vi "AIT 1553 - Read FIFOs.vi"(5 "Bus Section":T1, 7 "Mode":T2, 8 "error in (no error)":errorcluster, 11 "RT Data in":T3 {"Acyclic Frame Refs" format="%.0x"; "Label Transfer Config"."Block Data Refs"."Data Reference" format="%.0x"; "Status Config"."HWOut Dur Ref" format="%.0x"; "Status Config"."HWIn Dur Ref" format="%.0x"; "Status Config"."HWOut Count Ref" format="%.0x"; "Status Config"."HWIn Count Ref" format="%.0x"; "Status Config"."Error Data Ref" format="%.0x"; "HWOutput Channels"."Message Settings"."Driver Data"."First Word" min=8 max=31; "HWOutput Channels"."Message Settings"."Driver Data"."Num Bits" min=1 max=32; "HWOutput Channels"."Message Settings"."Driver Data"."Start Bit" min=8 max=31; "HWOutput Channels"."Message Settings"."Block Data Refs"."Data Reference" format="%.0x"; "HWInput Channels"."Message Settings"."Driver Data"."First Word" min=8 max=31; "HWInput Channels"."Message Settings"."Driver Data"."Num Bits" min=1 max=32; "HWInput Channels"."Message Settings"."Driver Data"."Start Bit" min=8 max=31; "HWInput Channels"."Message Settings"."Block Data Refs"."Data Reference" format="%.0x"}) -> (0 "error out":errorcluster, 3 "RT Data out":T3 {"Acyclic Frame Refs" format="%.0x"; "Label Transfer Config"."Block Data Refs"."Data Reference" format="%.0x"; "Status Config"."HWOut Dur Ref" format="%.0x"; "Status Config"."HWIn Dur Ref" format="%.0x"; "Status Config"."HWOut Count Ref" format="%.0x"; "Status Config"."HWIn Count Ref" format="%.0x"; "Status Config"."Error Data Ref" format="%.0x"; "HWOutput Channels"."Message Settings"."Driver Data"."First Word" min=8 max=31; "HWOutput Channels"."Message Settings"."Driver Data"."Num Bits" min=1 max=32; "HWOutput Channels"."Message Settings"."Driver Data"."Start Bit" min=8 max=31; "HWOutput Channels"."Message Settings"."Block Data Refs"."Data Reference" format="%.0x"; "HWInput Channels"."Message Settings"."Driver Data"."First Word" min=8 max=31; "HWInput Channels"."Message Settings"."Driver Data"."Num Bits" min=1 max=32; "HWInput Channels"."Message Settings"."Driver Data"."Start Bit" min=8 max=31; "HWInput Channels"."Message Settings"."Block Data Refs"."Data Reference" format="%.0x"})   [LabVIEW 2013, in "AIT 1553 Custom Device.lvlib"]
uses:
  AIT 1553 Custom Device.lvlib
  RT Controls/AIT 1553  - RT Data.ctl
  RT Controls/AIT 1553 - RT HW Channel.ctl
  RT Controls/AIT 1553 - Bus Section.ctl
  RT Controls/AIT 1553 - RT Message Settings.ctl
  <vilib>/NI Veristand/Custom Device API/Block Data Reference.ctl
  <vilib>/NI Veristand/Custom Device API/Data Reference.ctl
  RT Controls/AIT 1553 - Driver Data.ctl
  Controls and Global/Start Bit.ctl
  Controls and Global/Number of Bits.ctl
  RT Controls/AIT 1553 - Board Config Info.ctl
  RT Controls/AIT 1553 - Hardware Type.ctl
  RT Controls/Error Qs.ctl
  RT Controls/Status Channels Config.ctl
  RT Controls/FIFO.ctl
  RT Controls/Label Transfer Config.ctl
  <vilib>/NI Veristand/Custom Device API/Custom Device Item Ref.ctl
  RT Controls/ReadWrite Selector.ctl
  <vilib>/NI Veristand/Custom Device API/Custom Device API.lvlib
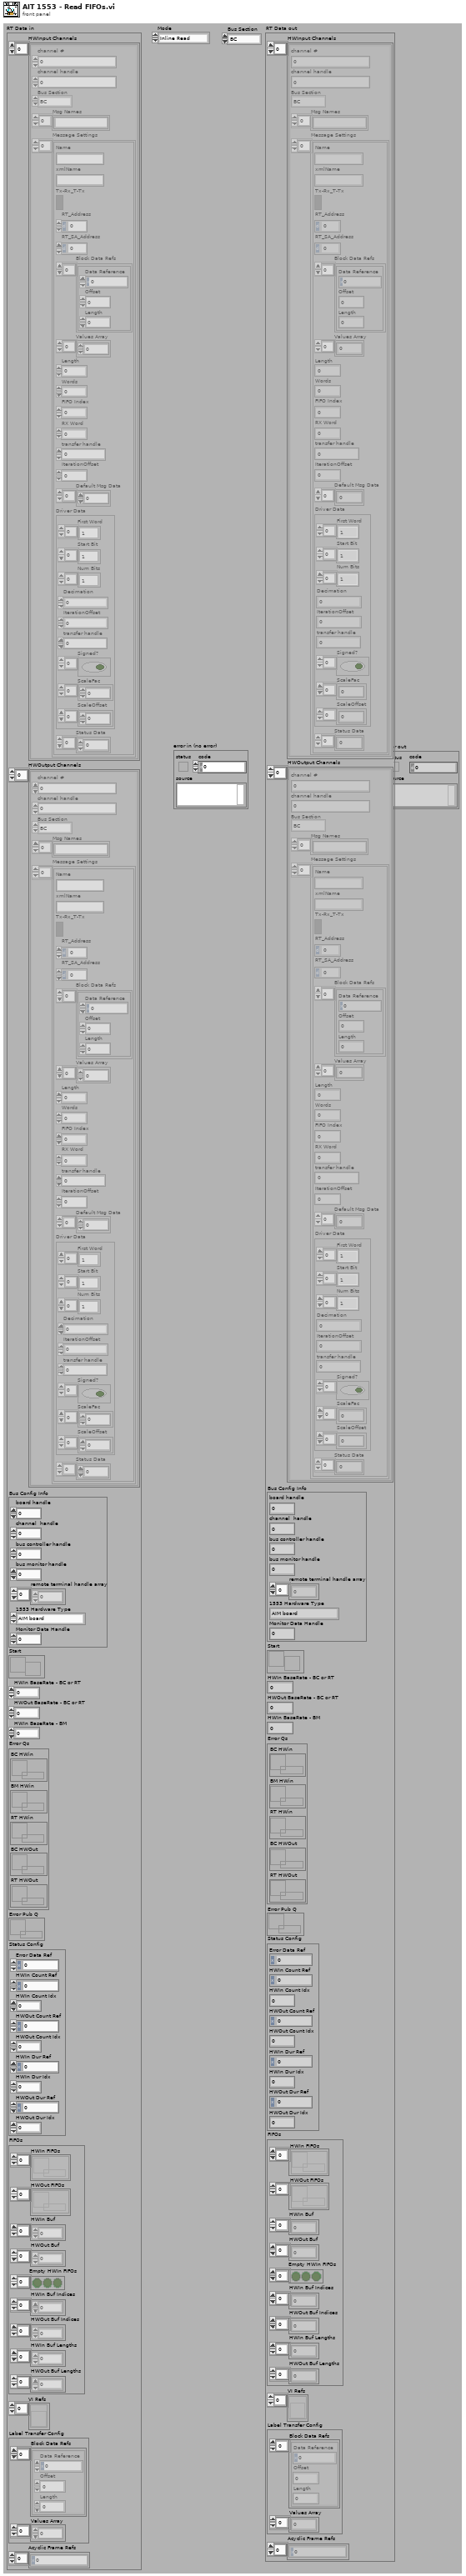
[diagram p1: front panel]
types:
  T1 = typedef "AIT 1553 Custom Device.lvlib/AIT 1553 - Bus Section.ctl" = enum16{"BC", "BM", "RT"}
  T2 = typedef "AIT 1553 Custom Device.lvlib/ReadWrite Selector.ctl" = enum16{"Inline Read", "Inline Write", "Async HWIn", "Async HWOut"}
  T3 = typedef "AIT 1553 Custom Device.lvlib/AIT 1553  - RT Data.ctl" = cluster{"HWInput Channels":T4[], "HWOutput Channels":T4[], "Bus Config Info":T11, "Start":refnum<notifier>, "HWIn BaseRate - BC or RT":i64, "HWOut BaseRate - BC or RT":i64, "HWIn BaseRate - BM":i64, "Error Qs":T13, "Error Pub Q":refnum<queue>, "Status Config":T14, "FIFOs":T15, "VI Refs":refnum<vi>[], "Label Transfer Config":T16, "Acyclic Frame Refs":T17[]}
  T4 = typedef "AIT 1553 Custom Device.lvlib/AIT 1553 - RT HW Channel.ctl" = cluster{"channel #":u16, "channel handle":u32, "Bus Section":T1, "Msg Names":string[], "Message Settings":T5[]}
  T5 = typedef "AIT 1553 Custom Device.lvlib/AIT 1553 - RT Message Settings.ctl" = cluster{"Name":string, "xmlName":string, "Tx-Rx_T-Tx":bool, "RT_Address":u8, "RT_SA_Address":u8, "Block Data Refs":T6[], "Values Array":dbl[], "Length":i32, "Words":i32, "FIFO Index":i32, "RX Word":u32, "transfer handle":u32, "IterationOffset":i32, "Default Msg Data":u16[], "Driver Data":T8, "Status Data":u32[]}
  T6 = typedef "Custom Device API.lvlib/Block Data Reference.ctl" = cluster{"Data Reference":T7, "Offset":i32, "Length":i32}
  T7 = typedef "Custom Device API.lvlib/Data Reference.ctl" = i32
  T8 = typedef "AIT 1553 Custom Device.lvlib/AIT 1553 - Driver Data.ctl" = cluster{"First Word":T9[], "Start Bit":T9[], "Num Bits":T10[], "Decimation":i32, "IterationOffset":i32, "transfer handle":u32, "Signed?":bool[], "ScaleFac":dbl[], "ScaleOffset":dbl[]}
  T9 = typedef "AIT 1553 Custom Device.lvlib/Start Bit.ctl" = i32
  T10 = typedef "AIT 1553 Custom Device.lvlib/Number of Bits.ctl" = i32
  T11 = typedef "AIT 1553 Custom Device.lvlib/AIT 1553 - Board Config Info.ctl" = cluster{"board handle":u32, "channel  handle":u32, "bus controller handle":u32, "bus monitor handle":u32, "remote terminal handle array":u32[], "1553 Hardware Type":T12, "Monitor Data Handle":u32}
  T12 = typedef "AIT 1553 Custom Device.lvlib/AIT 1553 - Hardware Type.ctl" = enum16{"AIM board", "AIT Board"}
  T13 = typedef "AIT 1553 Custom Device.lvlib/Error Qs.ctl" = cluster{"BC HWin":refnum<queue>, "BM HWin":refnum<queue>, "RT HWin":refnum<queue>, "BC HWOut":refnum<queue>, "RT HWOut":refnum<queue>}
  T14 = typedef "AIT 1553 Custom Device.lvlib/Status Channels Config.ctl" = cluster{"Error Data Ref":T7, "HWIn Count Ref":T7, "HWIn Count Idx":i32, "HWOut Count Ref":T7, "HWOut Count Idx":i32, "HWIn Dur Ref":T7, "HWIn Dur Idx":i32, "HWOut Dur Ref":T7, "HWOut Dur Idx":i32}
  T15 = typedef "AIT 1553 Custom Device.lvlib/FIFO.ctl" = cluster{"HWIn FIFOs":refnum<k33>[], "HWOut FIFOs":refnum<k33>[], "HWIn Buf":dbl[], "HWOut Buf":dbl[], "Empty HWIn FIFOs":bool[], "HWIn Buf Indices":i32[], "HWOut Buf Indices":i32[], "HWIn Buf Lengths":i32[], "HWOut Buf Lengths":i32[]}
  T16 = typedef "AIT 1553 Custom Device.lvlib/Label Transfer Config.ctl" = cluster{"Block Data Refs":T6[], "Values Array":dbl[]}
  T17 = typedef "Custom Device API.lvlib/Custom Device Item Ref.ctl" = u64
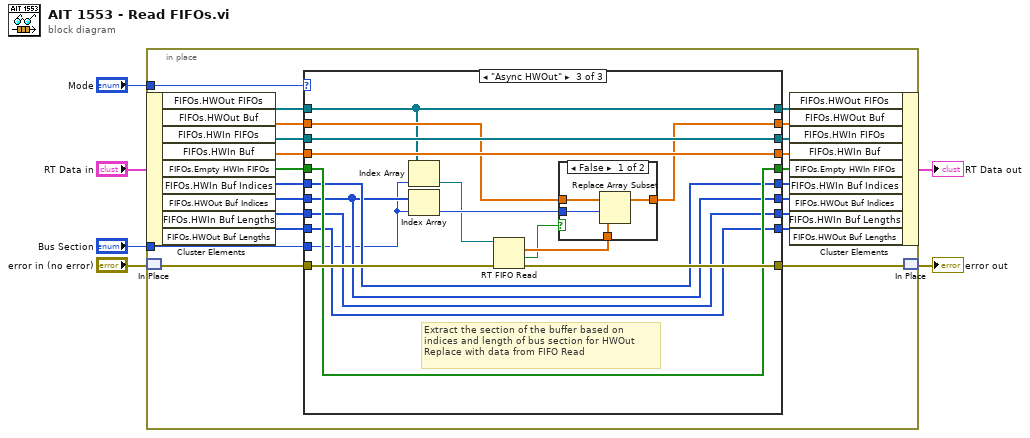
[diagram p0: block diagram]
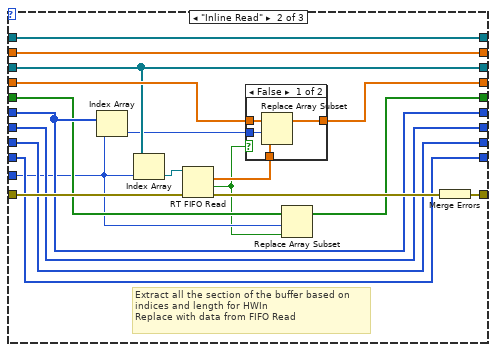
[diagram p3: hidden frame]
diagram:
  n1 = in-place {
    in-place-border: "Mode" -> [w21]
    in-place-border: "Bus Section" -> [w13]
    n2 = in-place-cluster #1("RT Data in") -> ("FIFOs.HWOut FIFOs"=w19:refnum<k33>[], "FIFOs.HWOut Buf"=w18:dbl[], "FIFOs.HWIn FIFOs"=w28:refnum<k33>[], "FIFOs.HWIn Buf"=w27:dbl[], "FIFOs.Empty HWIn FIFOs"=w20:bool[], "FIFOs.HWIn Buf Indices"=w12:i32[], "FIFOs.HWOut Buf Indices"=w15:i32[], "FIFOs.HWIn Buf Lengths"=w9:i32[], "FIFOs.HWOut Buf Lengths"=w14:i32[])
    n3 = in-place-match #2("error in (no error)") -> (w23:errorcluster)
    n4 = case shown="\"Async HWOut\"" w21 {
      tunnel: w28 -> [w37 w46 w76]
      tunnel: w27 -> [w38 w50 w77]
      tunnel: [w38 w48 w77] -> w26
      tunnel: [w37 w46 w76] -> w25
      tunnel: [w36 w39 w75] -> w24
      tunnel: w23 -> [w35 w57 w79]
      tunnel: [w35 w49 w78] -> w22
      tunnel: w20 -> [w36 w42 w75]
      tunnel: w19 -> [w33 w54 w66]
      tunnel: w18 -> [w34 w55 w74]
      tunnel: [w33 w54 w66] -> w17
      tunnel: [w34 w55 w71] -> w16
      tunnel: w15 -> [w31 w53 w69]
      tunnel: w14 -> [w29 w52 w67]
      tunnel: w13 -> [_ w41 w65]
      tunnel: [w32 w44 w70] -> w11
      tunnel: w12 -> [w32 w44 w70]
      tunnel: [w31 w53 w69] -> w10
      tunnel: [w30 w51 w68] -> w8
      tunnel: w9 -> [w30 w51 w68]
      tunnel: [w29 w52 w67] -> w7
      frame Default {
      }
      frame "Inline Read" {
        # "Extract all the section of the buffer based on \nindices and length for HWIn\nReplace with data from FIFO Read"
        n5 = Index Array(array=w44, index=w41) -> (element=w43:i32)
        n6 = Index Array(array=w46, index=w41) -> (element=w45:refnum<k33>)
        n7 = RT FIFO Read(0:w45, 3:w57) -> (9:w47:dbl[], 10:w40:bool, 11:w56:errorcluster)  [unwired: 2 in, 2 out]
        n8 = case shown="False" w40 {
          tunnel: w47 -> [w61 _]
          tunnel: w43 -> [w60 _]
          tunnel: w50 -> [w59 w62]
          tunnel: [w58 w62] -> w48
          frame False {
            n9 = Replace Array Subset(array=w59, new element=w61, index=w60) -> (w58:dbl[])
          }
          frame True {
          }
        }
        n10 = Replace Array Subset(array=w42, new element=w40, index=w41) -> (w39:bool[])
        n11 = Merge Errors(w56) -> (w49:errorcluster)
      }
      frame "Async HWOut" {
        # "Extract the section of the buffer based on \nindices and length of bus section for HWOut\nReplace with data from FIFO Read"
        n12 = Index Array(array=w66, index=w65) -> (element=w64:refnum<k33>)
        n13 = Index Array(array=w69, index=w65) -> (element=w73:i32)
        n14 = RT FIFO Read(0:w64, 3:w79) -> (9:w72:dbl[], 10:w63:bool, 11:w78:errorcluster)  [unwired: 2 in, 2 out]
        n15 = case shown="False" w63 {
          tunnel: w74 -> [w83 w84]
          tunnel: w73 -> [w82 _]
          tunnel: w72 -> [w81 _]
          tunnel: [w80 w84] -> w71
          frame False {
            n16 = Replace Array Subset(array=w83, new element=w81, index=w82) -> (w80:dbl[])
          }
          frame True {
          }
        }
      }
    }
    n17 = in-place-cluster #1("FIFOs.HWOut FIFOs"=w17, "FIFOs.HWOut Buf"=w16, "FIFOs.HWIn FIFOs"=w25, "FIFOs.HWIn Buf"=w26, "FIFOs.Empty HWIn FIFOs"=w24, "FIFOs.HWIn Buf Indices"=w11, "FIFOs.HWOut Buf Indices"=w10, "FIFOs.HWIn Buf Lengths"=w8, "FIFOs.HWOut Buf Lengths"=w7) -> (→"RT Data out":T3)
    n18 = in-place-match #2(w22) -> (→"error out":errorcluster)
  }
